vi "Solve1.vi"(8 "Error In":errorcluster, 11 "object in":refnum<class "2022_8.lvclass">) -> (0 "Error Out":errorcluster, 2 "Result":u64, 3 "object out":refnum<class "2022_8.lvclass">)   [LabVIEW 2020, in "2022_8.lvclass"]
uses:
  2022_8.lvclass
  2022_8.lvclass/2022_8.ctl
panel:
  out "Map":u8[][](array[numeric])
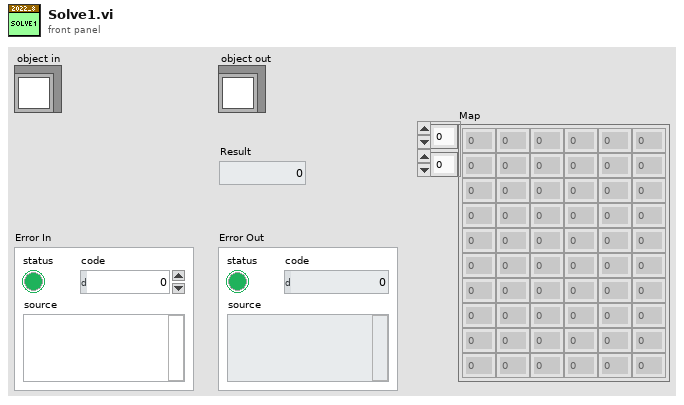
[diagram p1: front panel]
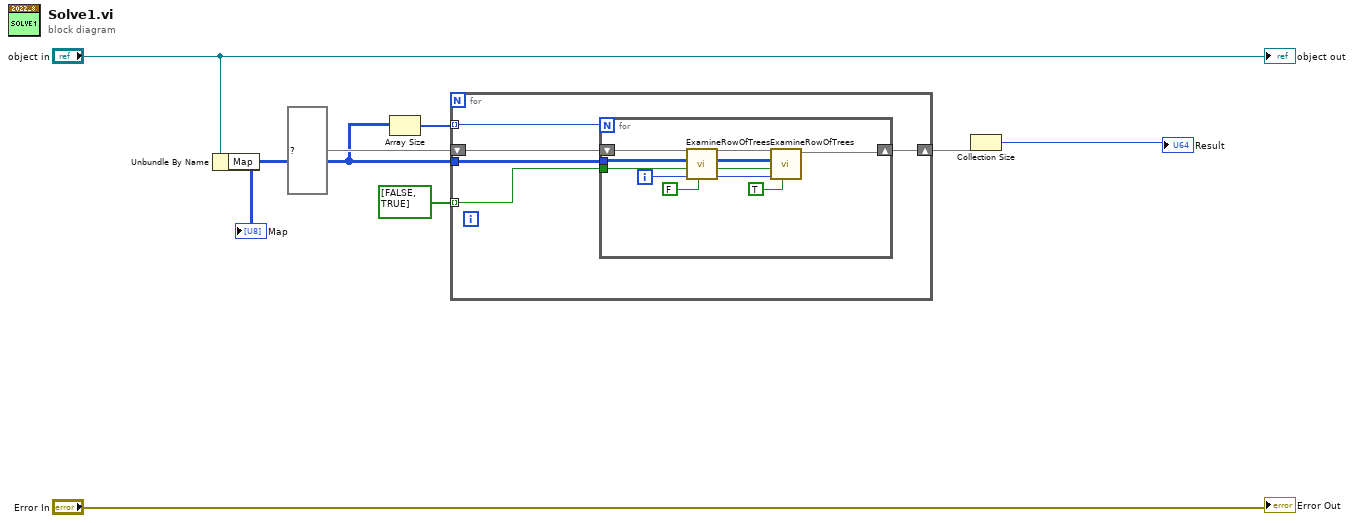
[diagram p0: block diagram]
diagram:
  n1 = Unbundle By Name("object in") -> ("Map"=w4:u8[][])
  "Map" <- w4
  n2 = Array Size(array=w4) -> (size(s)=w3:i32[])
  n3 = for {
    tunnel: w4 -> [w13]
    shift-right: [w11] -> w2
    shift-left: set{cluster{"Row":i32, "Column":i32}} {} ("TreesVisiableOut") -> [w12]
    tunnel: bool[] [FALSE, TRUE] ("Column") -> [w10] mode=indexing
    tunnel: w3 -> [w9] mode=indexing
    n4 = for {
      N: w9 -> [_]
      tunnel: w13 -> [w18]
      shift-right: [w19] -> w11
      shift-left: w12 -> [w21]
      tunnel: w10 -> [w14]
      i -> [w17]
      n5 = call "ExamineRowOfTrees.vi"("ReversSearchDirection"=FALSE, "Row/Column"=w17, "Column"=w14, "MapIn"=w18, "TreesVisiableIn"=w21) -> ("TreesVisiableOut"=w20:set{cluster{"Row":i32, "Column":i32}})  [unwired: 6 in]
      n6 = call "ExamineRowOfTrees.vi"("ReversSearchDirection"=TRUE, "Row/Column"=w17, "Column"=w14, "MapIn"=w18, "TreesVisiableIn"=w20) -> ("TreesVisiableOut"=w19:set{cluster{"Row":i32, "Column":i32}})  [unwired: 6 in]
    }
  }
  n7 = Collection Size(1:w2) -> (0:→"Result":i32)
  "Error Out" <- "Error In"
  "object out" <- "object in"
